vi "AS_IN.vi"(5 "掃碼L結果":string, 7 "掃碼R結果":string, 8 "error in (no error)":errorcluster, 9 "拍攝L讀取條碼":string, 10 "拍攝R讀取條碼":string, 11 "DBLink":string) -> (0 "error out":errorcluster, 3 "資料紀錄結果":string)   [LabVIEW 2019]
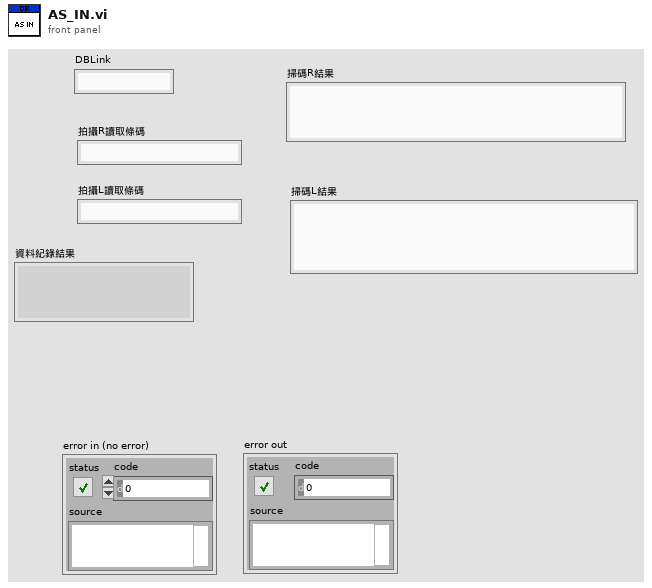
[diagram p1: front panel]
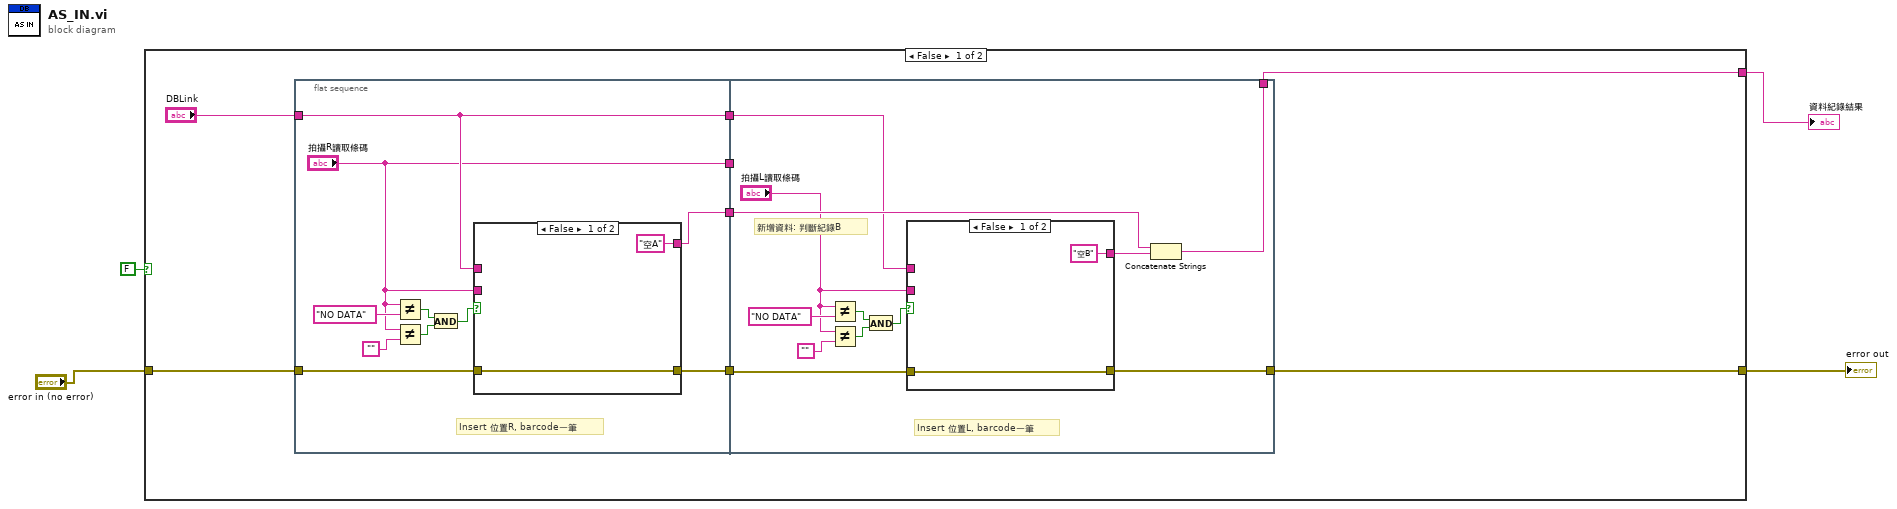
[diagram p0: block diagram]
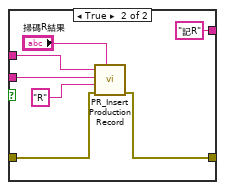
[diagram p2: hidden frame]
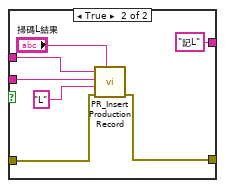
[diagram p3: hidden frame]
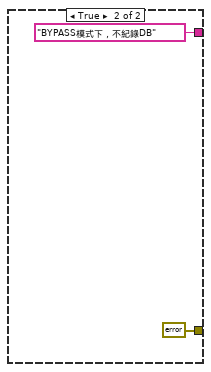
[diagram p4: hidden frame]
diagram:
  n1 = case shown="False" FALSE {
    tunnel: [w5 errorcluster {"status"=FALSE, "code"=0, "source"=""} ("error out")] -> w4
    tunnel: "error in (no error)" -> [w7 _]
    tunnel: [w6 "BYPASS模式下，不紀錄DB"] -> w2
    frame False {
      n2 = flat-sequence {
        tunnel: "DBLink" -> [w22]
        tunnel: [w22] -> w12
        tunnel: w7 -> [w21]
        tunnel: [w20] -> w11
        tunnel: [w19] -> w10
        tunnel: ["拍攝R讀取條碼"] -> w9
        tunnel: w12 -> [w40]
        tunnel: w11 -> [w43]
        tunnel: w10 -> [w42]
        tunnel: w9 -> [_]
        tunnel: [w39] -> w6
        tunnel: [w38] -> w5
        frame #0 {
          # "Insert 位置R, barcode一筆"
          n3 = Not Equal?(x="拍攝R讀取條碼", y="NO DATA") -> (x != y?=w14:bool)
          n4 = Not Equal?(x="拍攝R讀取條碼", y="") -> (x != y?=w15:bool)
          n5 = And(x=w14, y=w15) -> (x .and. y?=w13:bool)
          n6 = case shown="False" w13 {
            tunnel: w22 -> [_ w31]
            tunnel: "拍攝R讀取條碼" -> [_ w30]
            tunnel: w21 -> [w24 w28]
            tunnel: [w24 w27] -> w20
            tunnel: ["空A" "記R"] -> w19
            frame False {
            }
            frame True {
              n7 = call "PR_Insert Production Record.vi"("search_result"="掃碼R結果", "error in (no error)"=w28, "position"="R" ("pos"), "barcode"=w30, "DBlink"=w31) -> ("error out"=w27:errorcluster)  [unwired: 6 in]
            }
          }
        }
        frame #1 {
          # "Insert 位置L, barcode一筆"
          # "新增資料: 判斷紀錄B"
          n8 = Not Equal?(x="拍攝L讀取條碼", y="NO DATA") -> (x != y?=w34:bool)
          n9 = Not Equal?(x="拍攝L讀取條碼", y="") -> (x != y?=w35:bool)
          n10 = And(x=w34, y=w35) -> (x .and. y?=w32:bool)
          n11 = case shown="False" w32 {
            tunnel: w40 -> [_ w52]
            tunnel: "拍攝L讀取條碼" -> [_ w51]
            tunnel: [w44 w49] -> w38
            tunnel: ["空B" "記L"] -> w41
            tunnel: w43 -> [w44 w46]
            frame False {
            }
            frame True {
              n12 = call "PR_Insert Production Record.vi"("search_result"="掃碼L結果", "error in (no error)"=w46, "position"="L" ("pos"), "barcode"=w51, "DBlink"=w52) -> ("error out"=w49:errorcluster)  [unwired: 6 in]
            }
          }
          n13 = Concatenate Strings(w42, w41) -> (w39:string)
        }
      }
    }
    frame True {
    }
  }
  "error out" <- w4
  "資料紀錄結果" <- w2
